vi "FPGA.vi"() -> ()   [LabVIEW 2013]
uses:
  <vilib>/Platform/TimedLoop/XDataNode/timing_clust.ctl
  <vilib>/Platform/TimedLoop/XDataNode/nitl_modes.ctl
  <vilib>/Platform/TimedLoop/XDataNode/wakeup.ctl
  <vilib>/rvi/FXPMathLib/basic elements/FxpIntAccumulator/subVIs/nifxpmath_IntAccumulator_SimConfig.ctl
  <vilib>/rvi/Emulation/niFpgaSctlEmulationGetInTimedLoop.vi
  <vilib>/rvi/Emulation/niFpgaEmulationReportErrorSimple.vi
  <vilib>/rvi/Emulation/niFpgaGetClockAttributes.vi
  <vilib>/rvi/eio/common/nirviEmuTemplateMethod_errors.vi
  <vilib>/rvi/Emulation/niFpgaCriticalErrorInLSC.vi
  <vilib>/rvi/Emulation/niFpgaProcessEmulError.vi
  <vilib>/rvi/Analysis/common/codeGenErrors/XNode/niFpgaXNodeCodeGenErrorHandle.vi
  <vilib>/rvi/FXPMathLib/basic elements/FxpIntAccumulator/simVIs/DllFxpIntAccumulator_sub.vi
  <vilib>/eio/EIONode/EIONode.xnode
  <vilib>/LabVIEW Targets/FPGA/RIO/nicrio_985x_controls.llb/CAN_IO_Frame Cluster.ctl
  <vilib>/LabVIEW Targets/FPGA/RIO/nicrio_985x_controls.llb/CAN_IO_Frame Type.ctl
  <vilib>/rvi/Analysis/measure/dc-rms/XNode/niFpgaDC-RMS.xnode
  <vilib>/Platform/TimedLoop/XDataNode/XDataNode.xnode
  <vilib>/rvi/FXPMathLib/basic elements/FxpIntAccumulator/XNode/nifxpmath_IntAccumulator.xnode
  <vilib>/rvi/FXPMathLib/FxpMul/XNode/nifxpmath_Multiplier.xnode
  <vilib>/LabVIEW Targets/FPGA/RIO/nicrio_985x_controls.llb/CAN_IO_Frame Array U32.ctl
  <vilib>/rvi/Analysis/measure/butterworth/XNode/niFpgaButterworthFilter.xnode
  <vilib>/Platform/TimedLoop/XDataNode/XDNodeRunTimeDep.lvlib
  <vilib>/rvi/FXPMathLib/sim/FxpSim.dll
panel:
  out "Speed":fxp<+/-,60,18>
  out "OpticalSensor":fxp<+/-,26,5>
  out "TorquePermitted":fxp<+/-,64,40>
  out "TD1":fxp<+/-,26,5>
  out "TD2":fxp<+/-,26,5>
  out "TD3":fxp<+/-,26,5>
  out "TD4":fxp<+/-,26,5>
  out "TD5":fxp<+/-,26,5>
  out "TD6":fxp<+/-,26,5>
  out "TD7":fxp<+/-,26,5>
  out "TD8":fxp<+/-,26,5>
  out "TD9":fxp<+/-,26,5>
  out "TD10":fxp<+/-,26,5>
  out "TD11":fxp<+/-,26,5>
  out "TD12":fxp<+/-,26,5>
  out "TD13":fxp<+/-,26,5>
  out "TD14":fxp<+/-,26,5>
  out "TD15":fxp<+/-,26,5>
  out "TD16":fxp<+/-,26,5>
  out "TD17":fxp<+/-,26,5>
  out "TD18":fxp<+/-,26,5>
  out "TD19":fxp<+/-,26,5>
  out "TD20":fxp<+/-,26,5>
  out "CurrencyDetector":fxp<+/-,26,5>
  out "Brake Detector":fxp<+/-,26,5>
  out "电池过温":bool
  out "电池过温_Sent":bool
  out "8Bytes_Received":u8[](array[numeric])
  out "ID_Received":u32
  in  "PowerPermitted":fxp<+/-,32,8>=80.0
  in  "ErrorMonitoring?":bool
  in  "发送间隔(mSec)":u8=1 caption="Count(mSec)"
  in  "接收窗口(mSec)":u8=20 caption="Count(mSec)"
  out "0x333Byte7":u8 format="%.0b"
  out "DashSwitches":u8 format="%.0b"
  in  "CAN Input Wait?":bool
  in  "开水泵温度值":fxp<+/-,32,16>=60.0
  in  "刹车标定上限":fxp<+,32,16>=3.1199951171875
  in  "开风扇温度值":fxp<+,8,6>=45.0 format="%#_21g"
  out "AMS_fed":bool
  out "FanO?":bool
  out "PumpO?":bool
  in  "cBSPD":bool
  in  "cAMS":bool
  out "SHTD":bool
  in  "BRAKELO":bool
  in  "BUZZERO":bool
  in  "AIRNO":bool
  in  "AIRPO":bool
  in  "PREO":bool
  out "BSPD?":bool
  out "IMD?":bool
  in  "AMS":bool=TRUE
  in  "P":fxp<+,32,32>
  in  "SPD":fxp<+,32,32>
  in  "M":fxp<+,32,32>
  in  "MA":bool
  in  "BA":bool
  in  "Ready":bool
  in  "MC1TqSet_L":u8
  in  "MC1TqSet_H":u8
  in  "MC2TqSet_L":u8
  in  "MC2TqSet_H":u8
  in  "MCCmdByte":u8
  in  "BMCmdByte":u8
  out "SIG_ACC2":fxp<+/-,30,9>
  out "SIG_ACC1":fxp<+/-,30,9>
  out "SIG_BRAKE":fxp<+/-,30,9>
  out "PREC_fed":bool
  out "PREO_fed":bool
  out "50%？":bool
  out "80%？":bool
  out "SWT4?":bool
  out "SWT3?":bool
  out "Stop？":bool
  out "Start？":bool
  out "BatteryErrorRank":u8
  out "MotorErrorRank":u8
  out "AIRPO_fed":bool
  out "AIRPC_fed":bool
  out "AIRNC_fed":bool
  out "AIRNO_fed":bool
  out "BMCellVMin":fxp<+/-,32,16>
  out "BMCellVMax":fxp<+/-,32,16>
  out "BMTemMean":fxp<+/-,32,16>
  out "BMTemMax":fxp<+/-,32,16>
  out "BMTemMin":fxp<+/-,32,16>
  out "BMIdLimt":fxp<+/-,32,16>
  out "BMSStatus":u8
  out "BMSVolIs":fxp<+/-,32,16>
  out "BMSIbIs":fxp<+/-,32,16>
  out "SOCMean":fxp<+/-,32,16>
  out "LinFR":fxp<+/-,32,16>
  out "LinFL":fxp<+/-,32,16>
  out "LinRR":fxp<+/-,32,16>
  out "LinRL":fxp<+/-,32,16>
  out "W2":fxp<+,29,3>
  out "WP":fxp<+,29,3>
  out "AX":fxp<+,29,3>
  out "AY":fxp<+,29,3>
  out "AZ":fxp<+,29,3>
  out "Wr":fxp<+,29,3>
  out "ACC1":fxp<+,29,3>
  out "ACC2":fxp<+,29,3>
  out "BRK1":fxp<+,29,3>
  out "STR":fxp<+,29,3>
  out "MC2VinIs":fxp<+/-,32,16>
  out "MC2TemIs":fxp<+/-,32,16>
  out "MC2InvTemIs":fxp<+/-,32,16>
  out "MC2TqLimt":fxp<+/-,32,16>
  out "MC2Status":u8
  out "MC2SpIs":fxp<+/-,32,16>
  out "MC2TqIs":fxp<+/-,32,16>
  out "MC2ImIs":fxp<+/-,32,16>
  out "MC1VinIs":fxp<+/-,32,16>
  out "MC1TemIs":fxp<+/-,32,16>
  out "MC1InvTemIs":fxp<+/-,32,16>
  out "MC1TqLimt":fxp<+/-,32,16>
  out "MC1Status":u8
  out "MC1SpIs":fxp<+/-,32,16>
  out "MC1TqIs":fxp<+/-,32,16>
  out "MC1ImIs":fxp<+/-,32,16>
  out "PowerLimited":fxp<+/-,16,6>=1.0
  # "80kw功率限制"
  # "Test Display"
  # "标定部分"
  # "Digital I/O"
  # "CAN Sending"
  # "Analog Input"
  # "CAN Input"
  # "Motor Control"
  # "Battery Management System"
  # "Sensor Node"
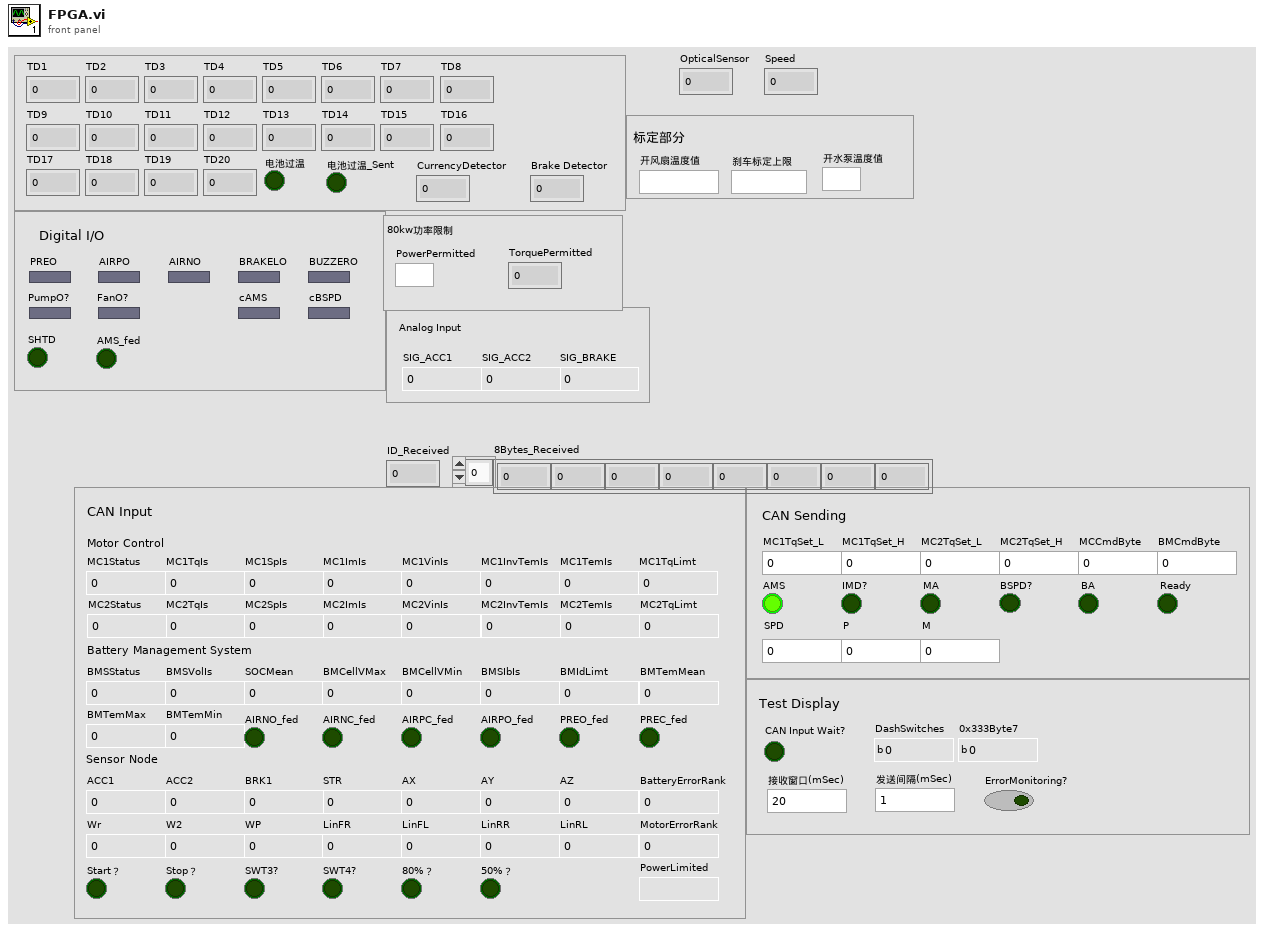
[diagram p1: front panel]
types:
  T1 = typedef "CAN_IO_Frame Cluster.ctl" = cluster{"timestamp high":u32, "timestamp low":u32, "identifier":u32, "type":T2, "info A":u8, "info B":u8, "data length":u8, "data":u8[]}
  T2 = typedef "CAN_IO_Frame Type.ctl" = enum8{"Data Frame", "Remote Frame", "(reserved)", "(reserved) ", "(reserved)  ", "(reserved)   ", "Bus Error", "Transceiver Fault"}
  T3 = typedef "XDNodeRunTimeDep.lvlib/timing_clust.ctl" = cluster{"Expected End [f-1]":u64, "Actual End [f-1]":u64, "Finished Late? [f-1]":bool, "Expected End [i-1]":u64, "Actual End [i-1]":u64, "Finished Late? [i-1]":bool, "Expected Start [i]":u64, "Actual Start [i]":u64, "Expected Start [f]":u64, "Actual Start [f]":u64, "Source Name":string, "Structure Name":string, "Period":i64, "Deadline":i64, "Offset":i64, "Start":i64, "Priority":i32, "Timeout":i32, "Mode":T4, "Wakeup Reason":T5, "Error":errorcluster, "Source Type":string, "Secondary Source Type":string, "Global End Time":u64, "Global Start Time":u64, "Frame Duration":u64, "Iteration Duration":u64, "Assigned CPU":i32, "I/O Scan Engine Mode":u32}
  T4 = typedef "XDNodeRunTimeDep.lvlib/nitl_modes.ctl" = enum32{"No Change", "Process missed periods, maintain original phase", "Discard missed periods, maintain original phase", "Process missed periods, ignore original phase", "Discard missed periods, ignore original phase"}
  T5 = typedef "XDNodeRunTimeDep.lvlib/wakeup.ctl" = enum32{"Normal", "Aborted", "Asynchronous wakeup", "Timing source error", "Timed loop error", "Timeout"}
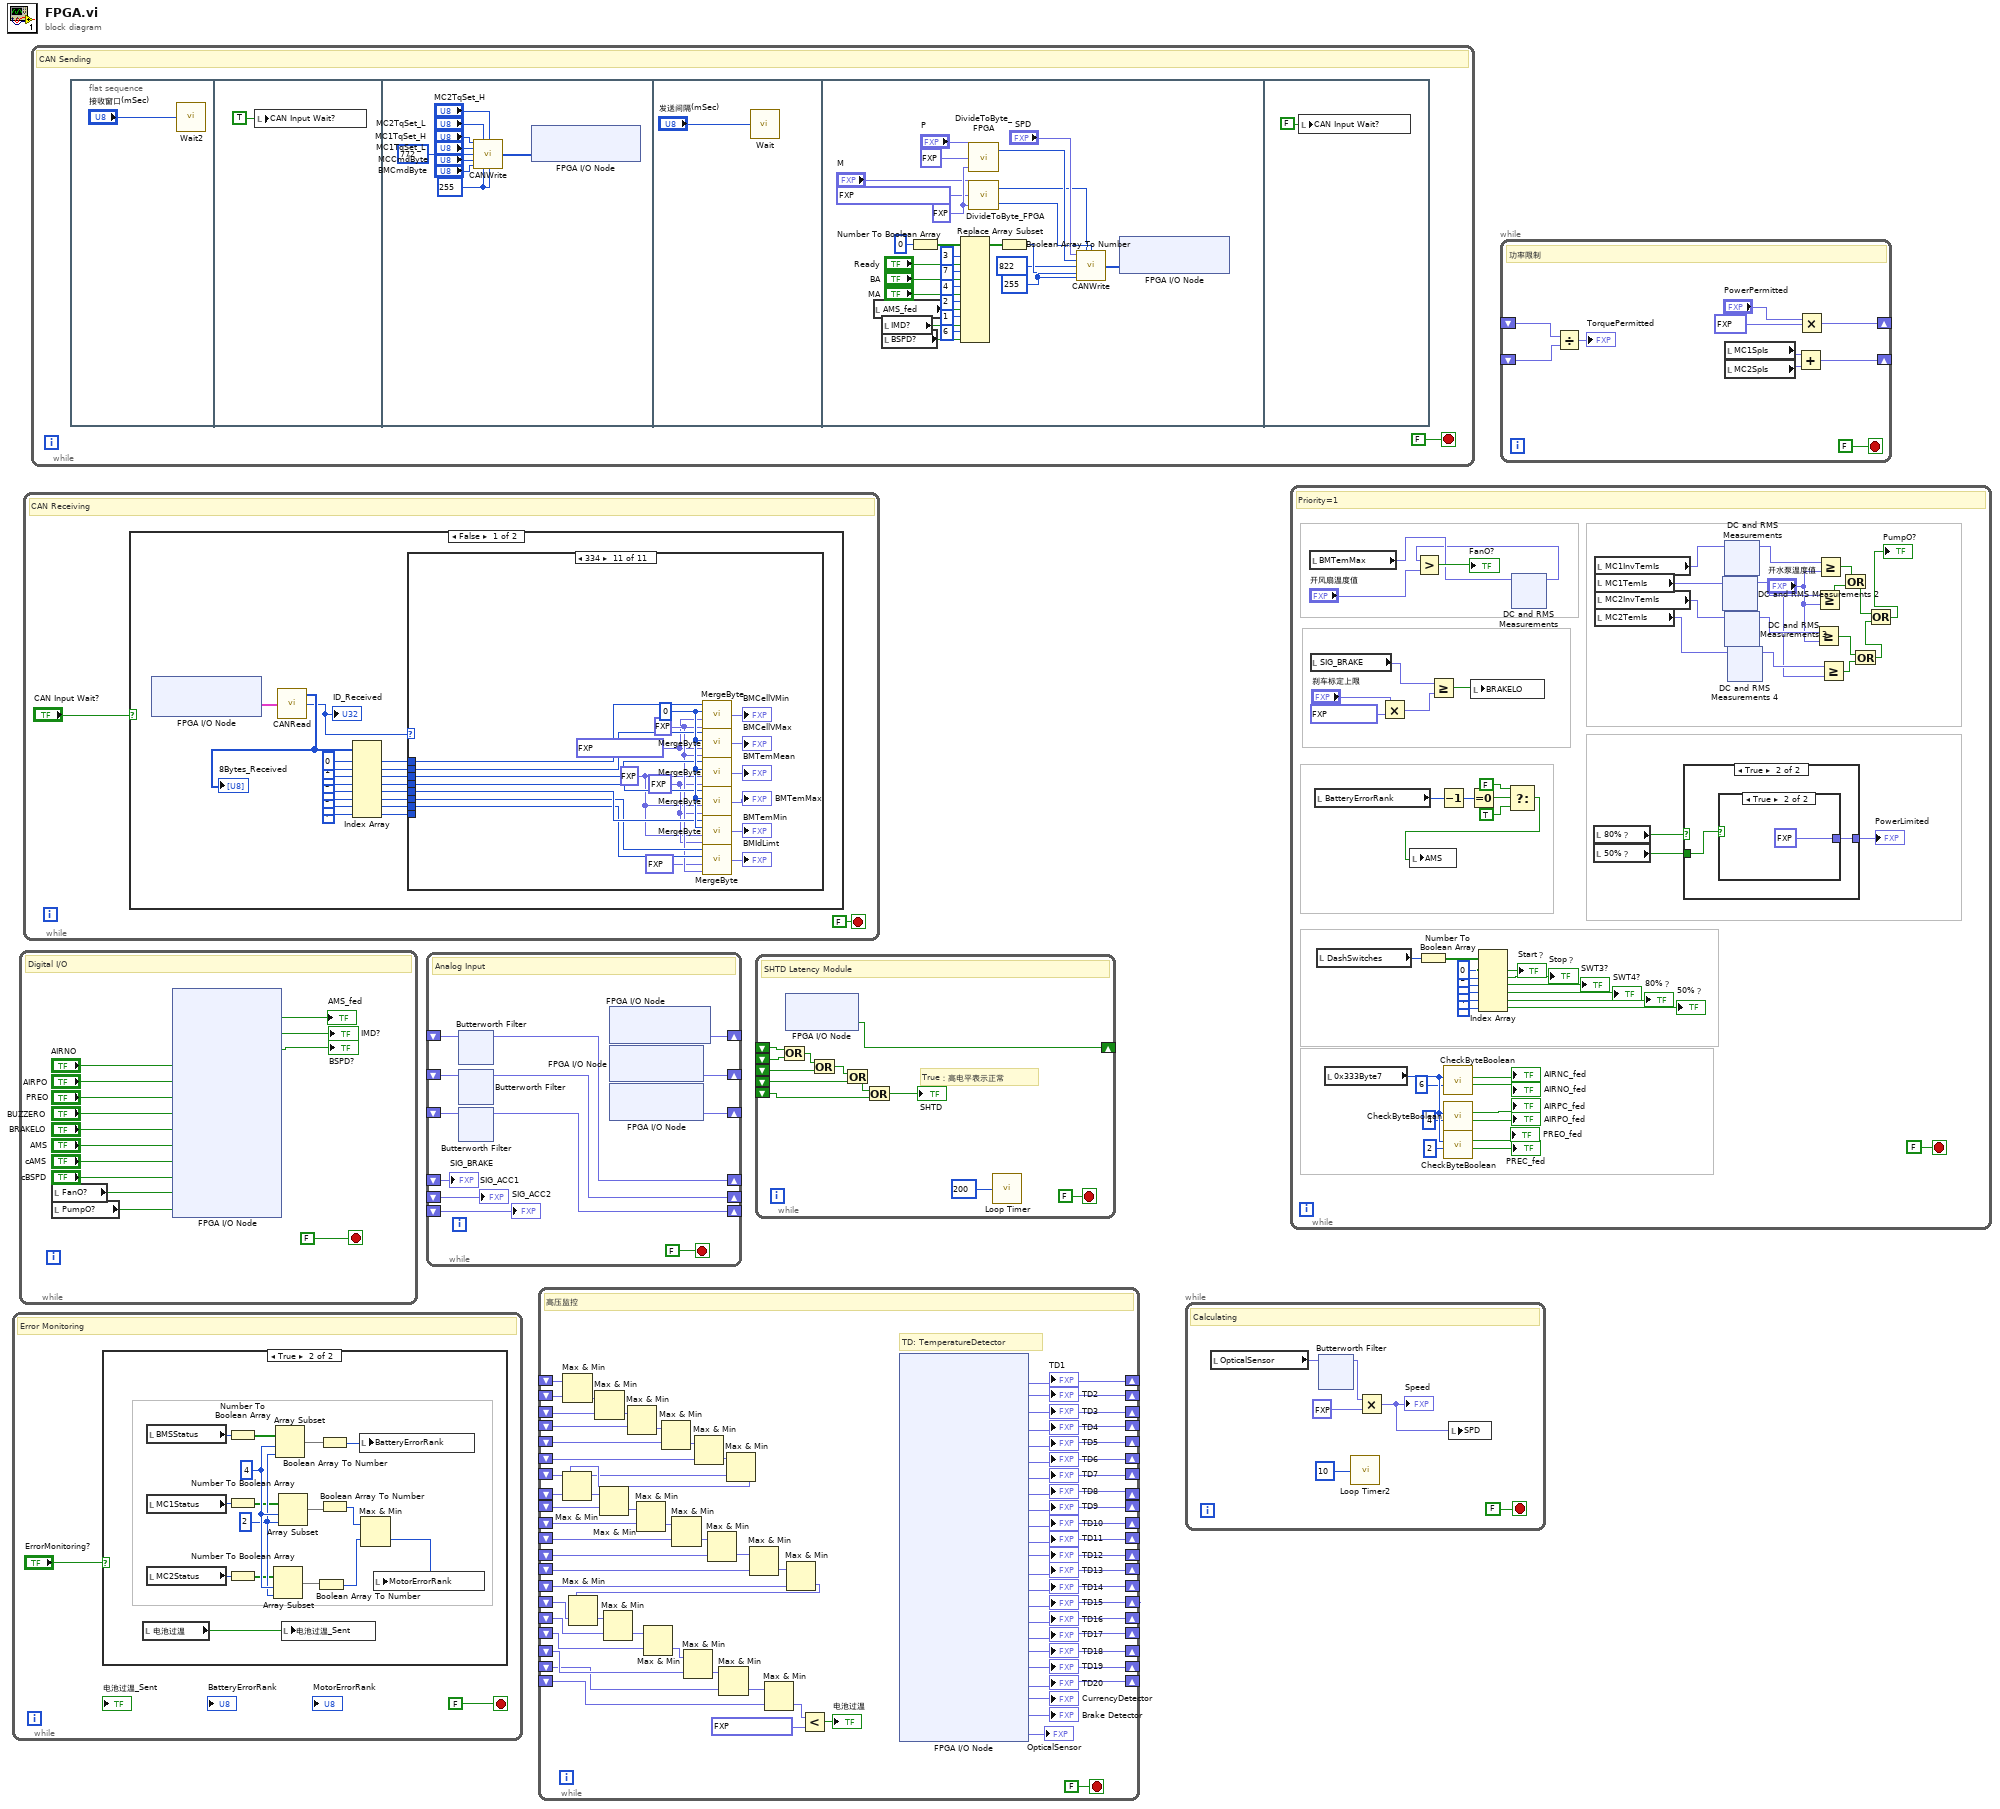
[diagram p0: block diagram]
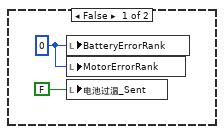
[diagram p2: hidden frame]
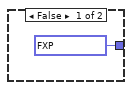
[diagram p3: hidden frame]
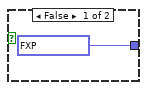
[diagram p4: hidden frame]
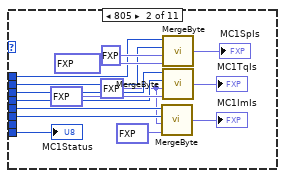
[diagram p6: hidden frame]
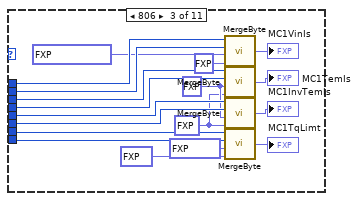
[diagram p7: hidden frame]
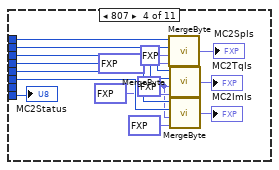
[diagram p8: hidden frame]
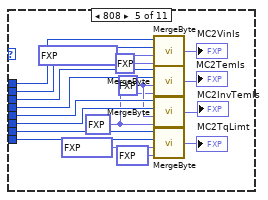
[diagram p9: hidden frame]
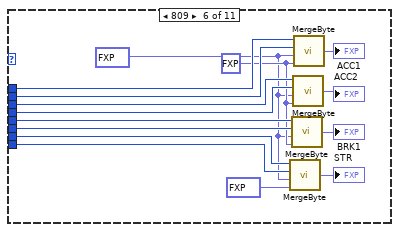
[diagram p10: hidden frame]
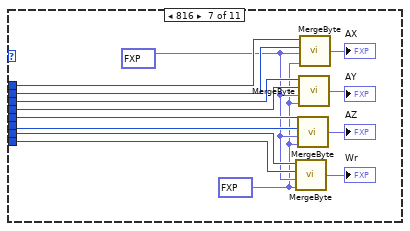
[diagram p11: hidden frame]
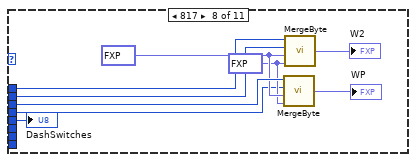
[diagram p12: hidden frame]
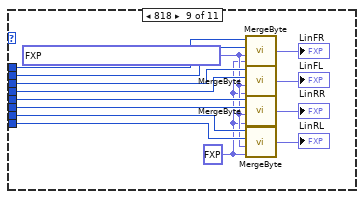
[diagram p13: hidden frame]
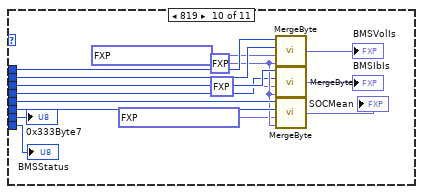
[diagram p14: hidden frame]
diagram:
  n1 = while {
    stop <- FALSE stop-if-true
    # "Error Monitoring"
    n2 = case shown="True" "ErrorMonitoring?" {
      frame False {
        w3 = u8 0 ("BatteryErrorRank")
        n3 = local write "BatteryErrorRank"(w3) -> ()
        n4 = local write "MotorErrorRank"(w3) -> ()
        n5 = local write "电池过温_Sent"(FALSE ("电池过温_Sent")) -> ()
      }
      frame True {
        w12 = 4 ("index")
        w11 = 2 ("length")
        n6 = local read "电池过温"() -> (w5:bool)
        n7 = local read "BMSStatus"() -> (w18:u8)
        n8 = local read "MC1Status"() -> (w19:u8)
        n9 = local read "MC2Status"() -> (w20:u8)
        n10 = Number To Boolean Array(number=w18) -> (Boolean array=w8:bool[])
        n11 = Number To Boolean Array(number=w19) -> (Boolean array=w9:bool[])
        n12 = Number To Boolean Array(number=w20) -> (Boolean array=w10:bool[])
        n13 = Array Subset(array=w10, index=w12, length=w11) -> (w15:bool[])
        n14 = Array Subset(array=w8, index=w12, length=w11) -> (w13:bool[])
        n15 = Array Subset(array=w9, index=w12, length=w11) -> (w14:bool[])
        n16 = local write "电池过温_Sent"(w5) -> ()
        n17 = Boolean Array To Number(Boolean array=w15) -> (number=w17:u8)
        n18 = Boolean Array To Number(Boolean array=w13) -> (number=w7:u8)
        n19 = Boolean Array To Number(Boolean array=w14) -> (number=w16:u8)
        n20 = local write "BatteryErrorRank"(w7) -> ()
        n21 = Max & Min(x=w16, y=w17) -> (min(x,y)=w6:u8)  [unwired: 1 out]
        n22 = local write "MotorErrorRank"(w6) -> ()
      }
    }
  }
  n23 = while {
    stop <- FALSE stop-if-true
    # "Digital I/O"
    n24 = local read "FanO?"() -> (w22:bool)
    n25 = local read "PumpO?"() -> (w23:bool)
    n26 = xnode "FPGA I/O Node"("AIRN"="AIRNO", "AIRP"="AIRPO", "PRE"="PREO", "BUZZER"="BUZZERO", "BRAKELED"="BRAKELO", "AMS_Sent"="AMS", "controlAMS"="cAMS", "controlBSPD"="cBSPD", "FAN"=w22, "PUM2"=w23) -> ("AMS"=→"AMS_fed":bool, "IMD"=→"IMD?":bool, "BSPD"=→"BSPD?":bool)  [unwired: 13 in, 13 out]
  }
  n27 = while {
    stop <- FALSE stop-if-true
    # "CAN Receiving"
    n28 = case shown="False" "CAN Input Wait?" {
      frame False {
        n29 = xnode "FPGA I/O Node"() -> ("Mod1/CAN0"=w55:T1)  [unwired: 2 in, 2 out]
        n30 = call "CANRead.vi"("CAN Signal"=w55) -> ("8Bytes_Received"=w54:u8[], "ID_Received"=w45:u32)  [unwired: 1 in]
        "ID_Received" <- w45
        "8Bytes_Received" <- w54
        n31 = Index Array(array=w54, index #1=0 ("index"), index #2=1 ("index"), index #3=2 ("index"), index #4=3 ("index"), index #5=4 ("index"), index #6=5 ("index"), index #7=6 ("index"), index #8=7 ("index")) -> (element #1=w44:u8, element #2=w43:u8, element #3=w42:u8, element #4=w41:u8, element #5=w40:u8, element #6=w39:u8, element #7=w38:u8, element #8=w37:u8)
        n32 = case shown="334" w45 {
          tunnel: w44 -> [_ w68 w88 w103 w121 w136 w146 w159 w173 w188 w206]
          tunnel: w43 -> [_ w67 w87 w102 w120 w135 w145 w158 w172 w187 w205]
          tunnel: w42 -> [_ w65 w86 w101 w119 w134 w144 w157 w171 w186 w204]
          tunnel: w41 -> [_ w64 w85 w100 w118 w133 w143 w152 w170 w175 w203]
          tunnel: w40 -> [_ w62 w84 w99 w117 w132 w142 w151 w169 w185 w202]
          tunnel: w39 -> [_ w61 w83 w98 w116 w131 w141 _ w168 w184 w201]
          tunnel: w38 -> [_ _ w82 _ w115 w130 w140 _ w167 w174 w200]
          tunnel: w37 -> [_ w60 w81 w97 w114 w129 w139 _ w166 w183 _]
          frame 0, Default {
          }
          frame 805 {
            w56 = fxp<+/-,32,16> 0.5 ("Resolution")
            n33 = call "MergeByte.vi"("Offset"=fxp<+/-,32,16> -200.0, "Resolution"=w56, "HighByte"=w61, "LowByte"=w62) -> ("Result"=→"MC1ImIs":fxp<+/-,32,16>)
            n34 = call "MergeByte.vi"("Offset"=fxp<+/-,32,16> -12000.0, "Resolution"=fxp<+/-,32,16> 1.0, "HighByte"=w67, "LowByte"=w68) -> ("Result"=→"MC1SpIs":fxp<+/-,32,16>)
            n35 = call "MergeByte.vi"("Offset"=fxp<+/-,32,16> -180.0, "Resolution"=w56, "HighByte"=w64, "LowByte"=w65) -> ("Result"=→"MC1TqIs":fxp<+/-,32,16>)
            "MC1Status" <- w60
          }
          frame 806 {
            w77 = fxp<+/-,32,16> -40.0 ("Offset")
            w78 = fxp<+/-,32,16> 1.0 ("Resolution")
            n36 = call "MergeByte.vi"("Offset"=fxp<+/-,32,16> 0.0, "Resolution"=fxp<+,8,-1> 0.349609375, "HighByte"=w87, "LowByte"=w88) -> ("Result"=→"MC1VinIs":fxp<+/-,32,16>)
            n37 = call "MergeByte.vi"("Offset"=w77, "Resolution"=w78, "HighByte"=w85, "LowByte"=w86) -> ("Result"=→"MC1TemIs":fxp<+/-,32,16>)
            n38 = call "MergeByte.vi"("Offset"=w77, "Resolution"=w78, "HighByte"=w83, "LowByte"=w84) -> ("Result"=→"MC1InvTemIs":fxp<+/-,32,16>)
            n39 = call "MergeByte.vi"("Offset"=fxp<+/-,32,16> -150.0, "Resolution"=fxp<+,5,-1> 0.40625, "HighByte"=w81, "LowByte"=w82) -> ("Result"=→"MC1TqLimt":fxp<+/-,32,16>)
          }
          frame 807 {
            w90 = fxp<+/-,32,16> 0.5 ("Resolution")
            n40 = call "MergeByte.vi"("Offset"=fxp<+/-,32,16> -12000.0, "Resolution"=fxp<+/-,32,16> 1.0, "HighByte"=w102, "LowByte"=w103) -> ("Result"=→"MC2SpIs":fxp<+/-,32,16>)
            n41 = call "MergeByte.vi"("Offset"=fxp<+/-,32,16> -150.0, "Resolution"=w90, "HighByte"=w100, "LowByte"=w101) -> ("Result"=→"MC2TqIs":fxp<+/-,32,16>)
            n42 = call "MergeByte.vi"("Offset"=fxp<+/-,32,16> -200.0, "Resolution"=w90, "HighByte"=w98, "LowByte"=w99) -> ("Result"=→"MC2ImIs":fxp<+/-,32,16>)
            "MC2Status" <- w97
          }
          frame 808 {
            w110 = fxp<+/-,32,16> -40.0 ("Offset")
            w111 = fxp<+/-,32,16> 1.0 ("Resolution")
            n43 = call "MergeByte.vi"("Offset"=fxp<+/-,32,16> 0.0, "Resolution"=fxp<+,8,-1> 0.349609375, "HighByte"=w120, "LowByte"=w121) -> ("Result"=→"MC2VinIs":fxp<+/-,32,16>)
            n44 = call "MergeByte.vi"("Offset"=w110, "Resolution"=w111, "HighByte"=w118, "LowByte"=w119) -> ("Result"=→"MC2TemIs":fxp<+/-,32,16>)
            n45 = call "MergeByte.vi"("Offset"=w110, "Resolution"=w111, "HighByte"=w116, "LowByte"=w117) -> ("Result"=→"MC2InvTemIs":fxp<+/-,32,16>)
            n46 = call "MergeByte.vi"("Offset"=fxp<+/-,32,16> -150.0, "Resolution"=fxp<+/-,32,16> 0.40625, "HighByte"=w114, "LowByte"=w115) -> ("Result"=→"MC2TqLimt":fxp<+/-,32,16>)
          }
          frame 809 {
            w124 = fxp<+/-,8,0> 0.0 ("Offset")
            w123 = fxp<+,32,30> 4095.0 ("Resolution")
            n47 = call "MergeByte.vi"("Offset"=fxp<+/-,32,16> 2048.0, "Resolution"=w123, "HighByte"=w129, "LowByte"=w130) -> ("Result"=→"STR":fxp<+/-,32,16>)
            n48 = call "MergeByte.vi"("Offset"=w124, "Resolution"=w123, "HighByte"=w131, "LowByte"=w132) -> ("Result"=→"BRK1":fxp<+/-,32,16>)
            n49 = call "MergeByte.vi"("Offset"=w124, "Resolution"=w123, "HighByte"=w133, "LowByte"=w134) -> ("Result"=→"ACC2":fxp<+/-,32,16>)
            n50 = call "MergeByte.vi"("Offset"=w124, "Resolution"=w123, "HighByte"=w135, "LowByte"=w136) -> ("Result"=→"ACC1":fxp<+/-,32,16>)
          }
          frame 816 {
            w137 = fxp<+/-,32,30> 2048.0 ("Offset")
            w138 = fxp<+,32,30> 4095.0 ("Resolution")
            n51 = call "MergeByte.vi"("Offset"=w137, "Resolution"=w138, "HighByte"=w139, "LowByte"=w140) -> ("Result"=→"Wr":fxp<+/-,32,16>)
            n52 = call "MergeByte.vi"("Offset"=w137, "Resolution"=w138, "HighByte"=w141, "LowByte"=w142) -> ("Result"=→"AZ":fxp<+/-,32,16>)
            n53 = call "MergeByte.vi"("Offset"=w137, "Resolution"=w138, "HighByte"=w143, "LowByte"=w144) -> ("Result"=→"AY":fxp<+/-,32,16>)
            n54 = call "MergeByte.vi"("Offset"=w137, "Resolution"=w138, "HighByte"=w145, "LowByte"=w146) -> ("Result"=→"AX":fxp<+/-,32,16>)
          }
          frame 817 {
            w153 = fxp<+/-,32,30> 2048.0 ("Offset")
            w156 = fxp<+,32,30> 4095.0 ("Resolution")
            n55 = call "MergeByte.vi"("Offset"=w153, "Resolution"=w156, "HighByte"=w152, "LowByte"=w157) -> ("Result"=→"WP":fxp<+/-,32,16>)
            n56 = call "MergeByte.vi"("Offset"=w153, "Resolution"=w156, "HighByte"=w158, "LowByte"=w159) -> ("Result"=→"W2":fxp<+/-,32,16>)
            "DashSwitches" <- w151
          }
          frame 818 {
            w164 = fxp<+/-,32,16> 0.0 ("Offset")
            w165 = fxp<+,24,-2> 0.0016113370656967163 ("Resolution")
            n57 = call "MergeByte.vi"("Offset"=w164, "Resolution"=w165, "HighByte"=w172, "LowByte"=w173) -> ("Result"=→"LinFR":fxp<+/-,32,16>)
            n58 = call "MergeByte.vi"("Offset"=w164, "Resolution"=w165, "HighByte"=w170, "LowByte"=w171) -> ("Result"=→"LinFL":fxp<+/-,32,16>)
            n59 = call "MergeByte.vi"("Offset"=w164, "Resolution"=w165, "HighByte"=w168, "LowByte"=w169) -> ("Result"=→"LinRR":fxp<+/-,32,16>)
            n60 = call "MergeByte.vi"("Offset"=w164, "Resolution"=w165, "HighByte"=w166, "LowByte"=w167) -> ("Result"=→"LinRL":fxp<+/-,32,16>)
          }
          frame 819 {
            w179 = fxp<+/-,32,16> 0.0 ("Offset")
            n61 = call "MergeByte.vi"("Offset"=w179, "Resolution"=fxp<+/-,32,16> 0.100006103515625, "HighByte"=w187, "LowByte"=w188) -> ("Result"=→"BMSVolIs":fxp<+/-,32,16>)
            n62 = call "MergeByte.vi"("Offset"=w179, "Resolution"=fxp<+/-,32,16> 0.5, "HighByte"=w175, "LowByte"=w186) -> ("Result"=→"BMSIbIs":fxp<+/-,32,16>)
            n63 = call "MergeByte.vi"("Offset"=w179, "Resolution"=fxp<+/-,32,16> 0.149993896484375, "HighByte"=w184, "LowByte"=w185) -> ("Result"=→"SOCMean":fxp<+/-,32,16>)
            "BMSStatus" <- w183
            "0x333Byte7" <- w174
          }
          frame 820 {
            w196 = fxp<+/-,32,16> 1.0 ("Resolution")
            w197 = fxp<+,6,-5> 0.02001953125 ("Resolution")
            w198 = fxp<+/-,32,16> -40.0 ("Offset")
            w199 = fxp<+/-,32,16> 0.0 ("Offset")
            w207 = u8 0 ("HighByte")
            n64 = call "MergeByte.vi"("Offset"=w199, "Resolution"=w197, "HighByte"=w207, "LowByte"=w206) -> ("Result"=→"BMCellVMin":fxp<+/-,32,16>)
            n65 = call "MergeByte.vi"("Offset"=w199, "Resolution"=w197, "HighByte"=w207, "LowByte"=w205) -> ("Result"=→"BMCellVMax":fxp<+/-,32,16>)
            n66 = call "MergeByte.vi"("Offset"=w198, "Resolution"=w196, "HighByte"=w207, "LowByte"=w204) -> ("Result"=→"BMTemMean":fxp<+/-,32,16>)
            n67 = call "MergeByte.vi"("Offset"=w198, "Resolution"=w196, "HighByte"=w207, "LowByte"=w203) -> ("Result"=→"BMTemMax":fxp<+/-,32,16>)
            n68 = call "MergeByte.vi"("Offset"=w198, "Resolution"=w196, "HighByte"=w207, "LowByte"=w202) -> ("Result"=→"BMTemMin":fxp<+/-,32,16>)
            n69 = call "MergeByte.vi"("Offset"=w199, "Resolution"=fxp<+/-,32,16> 0.25, "HighByte"=w200, "LowByte"=w201) -> ("Result"=→"BMIdLimt":fxp<+/-,32,16>)
          }
        }
      }
      frame True {
      }
    }
  }
  n70 = while {
    stop <- FALSE stop-if-true
    # "CAN Sending"
    n71 = flat-sequence {
      frame #0 {
        n72 = call "Wait2"("Count(mSec)"="接收窗口(mSec)") -> ()  [unwired: 1 out]
      }
      frame #1 {
        n73 = local write "CAN Input Wait?"(TRUE ("CAN Input Wait?")) -> ()
      }
      frame #2 {
        w211 = u8 255
        n74 = call "CANWrite.vi"("Data1"="MC1TqSet_H", "Data2"="MC2TqSet_L", "Data3"="MC2TqSet_H", "Data0"="MC1TqSet_L", "ID_ToSend"=u32 772, "Data4"="MCCmdByte", "Data5"="BMCmdByte", "Data6"=w211, "Data7"=w211) -> ("Frame"=w213:u32[])  [unwired: 6 in]
        n75 = xnode "FPGA I/O Node"("Mod1/CAN0"=w213) -> ()  [unwired: 1 in, 1 out]
      }
      frame #3 {
        n76 = call "Wait"("Count(mSec)"="发送间隔(mSec)") -> ()  [unwired: 1 out]
      }
      frame #4 {
        w245 = fxp<+/-,64,32> 0.0 ("Offset")
        w236 = u8 255 ("Data7")
        n77 = local read "AMS_fed"() -> (w246:bool)
        n78 = local read "IMD?"() -> (w247:bool)
        n79 = local read "BSPD?"() -> (w248:bool)
        n80 = Number To Boolean Array(number=u8 0) -> (Boolean array=w224:bool[])
        n81 = Replace Array Subset(array=w224, new element #1="Ready", index #1=u8 3 ("index"), new element #2="BA", index #2=u8 7 ("index"), new element #3="MA", index #3=u8 4 ("index"), new element #4=w246, index #4=u8 2 ("index"), new element #5=w247, index #5=u8 1 ("index"), new element #6=w248, index #6=u8 6 ("index")) -> (w225:bool[])
        n82 = call "DivideToByte_FPGA.vi"("Offset"=w245, "Resolution"=fxp<+/-,64,32> 0.5, "Value"="P") -> ("LowByte"=w242:u8)  [unwired: 1 out]
        n83 = call "DivideToByte_FPGA.vi"("Offset"=w245, "Resolution"=fxp<+/-,32,16> 0.100006103515625, "Value"="M") -> ("HighByte"=w238:u8, "LowByte"=w237:u8)
        n84 = Boolean Array To Number(Boolean array=w225) -> (number=w235:u8)
        n85 = call "CANWrite.vi"("Data1"="SPD", "Data2"=w237, "Data3"=w238, "Data0"=w242, "ID_ToSend"=u32 822, "Data4"=w235, "Data5"=w236, "Data6"=w236, "Data7"=w236) -> ("Frame"=w222:u32[])  [unwired: 6 in]
        n86 = xnode "FPGA I/O Node"("Mod1/CAN0"=w222) -> ()  [unwired: 1 in, 1 out]
      }
      frame #5 {
        n87 = local write "CAN Input Wait?"(FALSE ("CAN Input Wait?")) -> ()
      }
    }
  }
  n88 = while {
    shift-right: [w261] -> _
    shift-left: _ -> [w260]
    shift-right: [w259] -> _
    shift-left: _ -> [w258]
    shift-right: [w257] -> _
    shift-left: _ -> [w256]
    shift-right: [w255] -> _
    shift-left: _ -> [w252]
    shift-right: [w254] -> _
    shift-left: _ -> [w251]
    shift-right: [w253] -> _
    shift-left: _ -> [w250]
    stop <- FALSE stop-if-true
    # "Analog Input"
    n89 = xnode "Butterworth Filter"("input data"=w260) -> ("output data"=w255:fxp<+/-,30,9>)  [unwired: 2 in]
    n90 = xnode "Butterworth Filter"("input data"=w258) -> ("output data"=w254:fxp<+/-,30,9>)  [unwired: 2 in]
    n91 = xnode "Butterworth Filter"("input data"=w256) -> ("output data"=w253:fxp<+/-,30,9>)  [unwired: 2 in]
    n92 = xnode "FPGA I/O Node"() -> ("SIG_BRAKE"=w261:fxp<+/-,26,5>)  [unwired: 1 in, 1 out]
    n93 = xnode "FPGA I/O Node"() -> ("SIG_ACC1"=w259:fxp<+/-,26,5>)  [unwired: 1 in, 1 out]
    n94 = xnode "FPGA I/O Node"() -> ("SIG_ACC2"=w257:fxp<+/-,26,5>)  [unwired: 1 in, 1 out]
    "SIG_BRAKE" <- w252
    "SIG_ACC1" <- w251
    "SIG_ACC2" <- w250
  }
  n95 = while {
    shift-right: [w348] -> _
    shift-left: _ -> [w328]
    shift-right: [w347] -> _
    shift-left: _ -> [w327]
    shift-right: [w346] -> _
    shift-left: _ -> [w325]
    shift-right: [w345] -> _
    shift-left: _ -> [w312]
    shift-right: [w344] -> _
    shift-left: _ -> [w311]
    shift-right: [w343] -> _
    shift-left: _ -> [w310]
    shift-right: [w342] -> _
    shift-left: _ -> [w309]
    shift-right: [w341] -> _
    shift-left: _ -> [w308]
    shift-right: [w340] -> _
    shift-left: _ -> [w307]
    shift-right: [w339] -> _
    shift-left: _ -> [w306]
    shift-right: [w338] -> _
    shift-left: _ -> [w305]
    shift-right: [w337] -> _
    shift-left: _ -> [w304]
    shift-right: [w336] -> _
    shift-left: _ -> [w303]
    shift-right: [w335] -> _
    shift-left: _ -> [w301]
    shift-right: [w334] -> _
    shift-left: _ -> [w298]
    shift-right: [w333] -> _
    shift-left: _ -> [w297]
    shift-right: [w332] -> _
    shift-left: _ -> [w295]
    shift-right: [w331] -> _
    shift-left: _ -> [w293]
    shift-right: [w330] -> _
    shift-left: _ -> [w291]
    shift-right: [w329] -> _
    shift-left: _ -> [w289]
    stop <- FALSE stop-if-true
    # "TD: TemperatureDetector"
    # "高压监控"
    n96 = Max & Min(x=w328, y=w327) -> (min(x,y)=w326:fxp<+/-,26,5>)  [unwired: 1 out]
    n97 = Max & Min(x=w326, y=w325) -> (min(x,y)=w313:fxp<+/-,26,5>)  [unwired: 1 out]
    n98 = Max & Min(x=w313, y=w312) -> (min(x,y)=w324:fxp<+/-,26,5>)  [unwired: 1 out]
    n99 = Max & Min(x=w324, y=w311) -> (min(x,y)=w323:fxp<+/-,26,5>)  [unwired: 1 out]
    n100 = Max & Min(x=w323, y=w310) -> (min(x,y)=w322:fxp<+/-,26,5>)  [unwired: 1 out]
    n101 = Max & Min(x=w322, y=w309) -> (min(x,y)=w321:fxp<+/-,26,5>)  [unwired: 1 out]
    n102 = Max & Min(x=w321, y=w308) -> (min(x,y)=w320:fxp<+/-,26,5>)  [unwired: 1 out]
    n103 = Max & Min(x=w320, y=w307) -> (min(x,y)=w319:fxp<+/-,26,5>)  [unwired: 1 out]
    n104 = Max & Min(x=w319, y=w306) -> (min(x,y)=w318:fxp<+/-,26,5>)  [unwired: 1 out]
    n105 = Max & Min(x=w318, y=w305) -> (min(x,y)=w317:fxp<+/-,26,5>)  [unwired: 1 out]
    n106 = Max & Min(x=w317, y=w304) -> (min(x,y)=w316:fxp<+/-,26,5>)  [unwired: 1 out]
    n107 = Max & Min(x=w316, y=w303) -> (min(x,y)=w302:fxp<+/-,26,5>)  [unwired: 1 out]
    n108 = Max & Min(x=w302, y=w301) -> (min(x,y)=w300:fxp<+/-,26,5>)  [unwired: 1 out]
    n109 = Max & Min(x=w300, y=w298) -> (min(x,y)=w299:fxp<+/-,26,5>)  [unwired: 1 out]
    n110 = Max & Min(x=w299, y=w297) -> (min(x,y)=w296:fxp<+/-,26,5>)  [unwired: 1 out]
    n111 = Max & Min(x=w296, y=w295) -> (min(x,y)=w294:fxp<+/-,26,5>)  [unwired: 1 out]
    n112 = Max & Min(x=w294, y=w293) -> (min(x,y)=w292:fxp<+/-,26,5>)  [unwired: 1 out]
    n113 = Max & Min(x=w292, y=w291) -> (min(x,y)=w290:fxp<+/-,26,5>)  [unwired: 1 out]
    n114 = Max & Min(x=w290, y=w289) -> (min(x,y)=w288:fxp<+/-,26,5>)  [unwired: 1 out]
    n115 = Less?(x=w288, y=fxp<+/-,16,2> 0.9912109375) -> (x < y?=→"电池过温":bool)
    n116 = xnode "FPGA I/O Node"() -> ("TD1"=w348:fxp<+/-,26,5>, "TD2"=w347:fxp<+/-,26,5>, "TD3"=w346:fxp<+/-,26,5>, "TD4"=w345:fxp<+/-,26,5>, "TD5"=w344:fxp<+/-,26,5>, "TD6"=w343:fxp<+/-,26,5>, "TD7"=w342:fxp<+/-,26,5>, "TD8"=w341:fxp<+/-,26,5>, "TD9"=w340:fxp<+/-,26,5>, "TD10"=w339:fxp<+/-,26,5>, "TD11"=w338:fxp<+/-,26,5>, "TD12"=w337:fxp<+/-,26,5>, "TD13"=w336:fxp<+/-,26,5>, "TD14"=w335:fxp<+/-,26,5>, "TD15"=w334:fxp<+/-,26,5>, "TD16"=w333:fxp<+/-,26,5>, "TD17"=w332:fxp<+/-,26,5>, "TD18"=w331:fxp<+/-,26,5>, "TD19"=w330:fxp<+/-,26,5>, "TD20"=w329:fxp<+/-,26,5>, "CurrentDetector"=→"CurrencyDetector":fxp<+/-,26,5>, "BrakeDetector"=→"Brake Detector":fxp<+/-,26,5>, "OpticalSensor"=→"OpticalSensor":fxp<+/-,26,5>)  [unwired: 23 in, 23 out]
    "TD1" <- w348
    "TD2" <- w347
    "TD3" <- w346
    "TD4" <- w345
    "TD5" <- w344
    "TD6" <- w343
    "TD7" <- w342
    "TD8" <- w341
    "TD9" <- w340
    "TD10" <- w339
    "TD11" <- w338
    "TD12" <- w337
    "TD13" <- w336
    "TD14" <- w335
    "TD15" <- w334
    "TD16" <- w333
    "TD17" <- w332
    "TD18" <- w331
    "TD19" <- w330
    "TD20" <- w329
  }
  n117 = while {
    shift-right: [w362] -> _
    shift-left: _ -> [w361]
    shift-left: _ -> [w360]
    shift-left: _ -> [w358]
    shift-left: _ -> [w356]
    shift-left: _ -> [w355]
    stop <- FALSE stop-if-true
    # "True：高电平表示正常"
    # "SHTD Latency Module"
    n118 = Or(x=w361, y=w360) -> (x .or. y?=w359:bool)
    n119 = xnode "FPGA I/O Node"() -> ("SHTD"=w362:bool)  [unwired: 1 in, 1 out]
    n120 = Or(x=w359, y=w358) -> (x .or. y?=w357:bool)
    n121 = Or(x=w357, y=w356) -> (x .or. y?=w354:bool)
    n122 = Or(x=w354, y=w355) -> (x .or. y?=→"SHTD":bool)
    n123 = call "Loop Timer"("Count(mSec)"=u8 200) -> ()  [unwired: 1 out]
  }
  n124 = while {
    stop <- FALSE stop-if-true
    # "Calculating"
    n125 = local read "OpticalSensor"() -> (w368:fxp<+/-,26,5>)
    n126 = xnode "Butterworth Filter"("input data"=w368) -> ("output data"=w367:fxp<+/-,30,9>)  [unwired: 2 in]
    n127 = call "Loop Timer2"("Count(mSec)"=u8 10) -> ()  [unwired: 1 out]
    n128 = Multiply(x=w367, y=fxp<+/-,30,9> 25.0) -> (x*y=w366:fxp<+/-,60,18>)
    "Speed" <- w366
    n129 = local write "SPD"(w366) -> ()
  }
  n130 = while {
    stop <- FALSE stop-if-true
    # "Priority=1"
    n131 = local read "BMTemMax"() -> (w386:fxp<+/-,32,16>)
    n132 = local read "SIG_BRAKE"() -> (w406:fxp<+/-,30,9>)
    n133 = local read "BatteryErrorRank"() -> (w384:u8)
    n134 = local read "DashSwitches"() -> (w418:u8)
    n135 = local read "0x333Byte7"() -> (w417:u8)
    n136 = Multiply(x="刹车标定上限", y=fxp<+,8,-1> 0.44921875) -> (x*y=w403:fxp<+,40,15>)
    n137 = Number To Boolean Array(number=w418) -> (Boolean array=w419:bool[])
    n138 = Greater Or Equal?(x=w406, y=w403) -> (x >= y?=w402:bool)
    n139 = Decrement(x=w384) -> (x-1=w383:u8)
    n140 = call "CheckByteBoolean.vi"("SingleByte"=w417, "StartIndex"=u8 6) -> ("=10？"=→"AIRNC_fed":bool, "=01？"=→"AIRNO_fed":bool)  [unwired: 6 in]
    n141 = call "CheckByteBoolean.vi"("SingleByte"=w417, "StartIndex"=u8 4) -> ("=10？"=→"AIRPC_fed":bool, "=01？"=→"AIRPO_fed":bool)  [unwired: 6 in]
    n142 = call "CheckByteBoolean.vi"("SingleByte"=w417, "StartIndex"=u8 2) -> ("=10？"=→"PREO_fed":bool, "=01？"=→"PREC_fed":bool)  [unwired: 6 in]
    n143 = Equal To 0?(x=w383) -> (x = 0?=w382:bool)
    n144 = local write "BRAKELO"(w402) -> ()
    n145 = Index Array(array=w419, index #1=0 ("index"), index #2=1 ("index"), index #3=2 ("index"), index #4=3 ("index"), index #5=4 ("index"), index #6=5 ("index")) -> (element #1=→"Start？":bool, element #2=→"Stop？":bool, element #3=→"SWT3?":bool, element #4=→"SWT4?":bool, element #5=→"80%？":bool, element #6=→"50%？":bool)
    n146 = Select(t=FALSE, s=w382, f=TRUE) -> (s? t:f=w379:bool)
    n147 = local write "AMS"(w379) -> ()
    n148 = xnode "DC and RMS Measurements"("input data"=w386) -> ("DC"=w385:fxp<+/-,32,16>)  [unwired: 1 in, 1 out]
    n149 = Greater?(x=w385, y="开风扇温度值") -> (0:→"FanO?":bool)
    n150 = local read "80%？"() -> (w433:bool)
    n151 = local read "50%？"() -> (w432:bool)
    n152 = local read "MC1InvTemIs"() -> (w401:fxp<+/-,32,16>)
    n153 = local read "MC1TemIs"() -> (w400:fxp<+/-,32,16>)
    n154 = local read "MC2InvTemIs"() -> (w399:fxp<+/-,32,16>)
    n155 = local read "MC2TemIs"() -> (w398:fxp<+/-,32,16>)
    n156 = case shown="True" w433 {
      tunnel: w432 -> [_ w839]
      tunnel: [fxp<+,8,0> 0.99609375 ("功率限制百分比") w838] -> w434
      frame False {
      }
      frame True {
        n157 = case shown="True" w839 {
          tunnel: [fxp<+,8,0> 0.80078125 ("功率限制百分比") fxp<+,8,0> 0.5 ("功率限制百分比")] -> w838
          frame False {
          }
          frame True {
          }
        }
      }
    }
    "PowerLimited" <- w434
    n158 = xnode ("DC and RMS Measurements 2")("input data"=w400) -> ("DC"=w396:fxp<+/-,32,16>)  [unwired: 1 in, 1 out]
    n159 = xnode ("DC and RMS Measurements")("input data"=w401) -> ("DC"=w397:fxp<+/-,32,16>)  [unwired: 1 in, 1 out]
    n160 = xnode ("DC and RMS Measurements 3")("input data"=w399) -> ("DC"=w395:fxp<+/-,32,16>)  [unwired: 1 in, 1 out]
    n161 = xnode ("DC and RMS Measurements 4")("input data"=w398) -> ("DC"=w394:fxp<+/-,32,16>)  [unwired: 1 in, 1 out]
    n162 = Greater Or Equal?(x=w395, y="开水泵温度值") -> (x >= y?=w390:bool)
    n163 = Greater Or Equal?(x=w396, y="开水泵温度值") -> (x >= y?=w392:bool)
    n164 = Greater Or Equal?(x=w397, y="开水泵温度值") -> (x >= y?=w393:bool)
    n165 = Greater Or Equal?(x=w394, y="开水泵温度值") -> (x >= y?=w391:bool)
    n166 = Or(x=w393, y=w392) -> (x .or. y?=w389:bool)
    n167 = Or(x=w390, y=w391) -> (x .or. y?=w388:bool)
    n168 = Or(x=w389, y=w388) -> (x .or. y?=→"PumpO?":bool)
  }
  n169 = while {
    shift-right: [w846] -> _
    shift-left: _ -> [w844]
    shift-right: [w845] -> _
    shift-left: _ -> [w843]
    stop <- FALSE stop-if-true
    # "功率限制"
    n170 = Divide(x=w844, y=w843) -> (x/y=→"TorquePermitted":fxp<+/-,64,40>)
    n171 = local read "MC1SpIs"() -> (w848:fxp<+/-,32,16>)
    n172 = local read "MC2SpIs"() -> (w849:fxp<+/-,32,16>)
    n173 = Add(x=w848, y=w849) -> (x+y=w845:fxp<+/-,33,17>)
    n174 = Multiply(x="PowerPermitted", y=fxp<+,16,16> 9550.0) -> (x*y=w846:fxp<+/-,48,24>)
  }
